vi "Alarm Playlist.vi"() -> ()   [LabVIEW 2011]
panel:
  in  "stop 3":bool
  out "Thief Alarm 2":bool
  in  "stop 2":bool
  out "Thief Alarm":bool
  in  "stop":bool
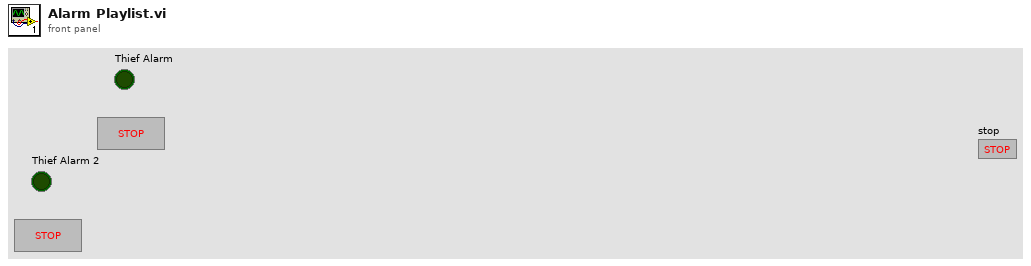
[diagram p1: front panel]
types:
  T1 = typedef "Sound Output Task ID.ctl" = u32
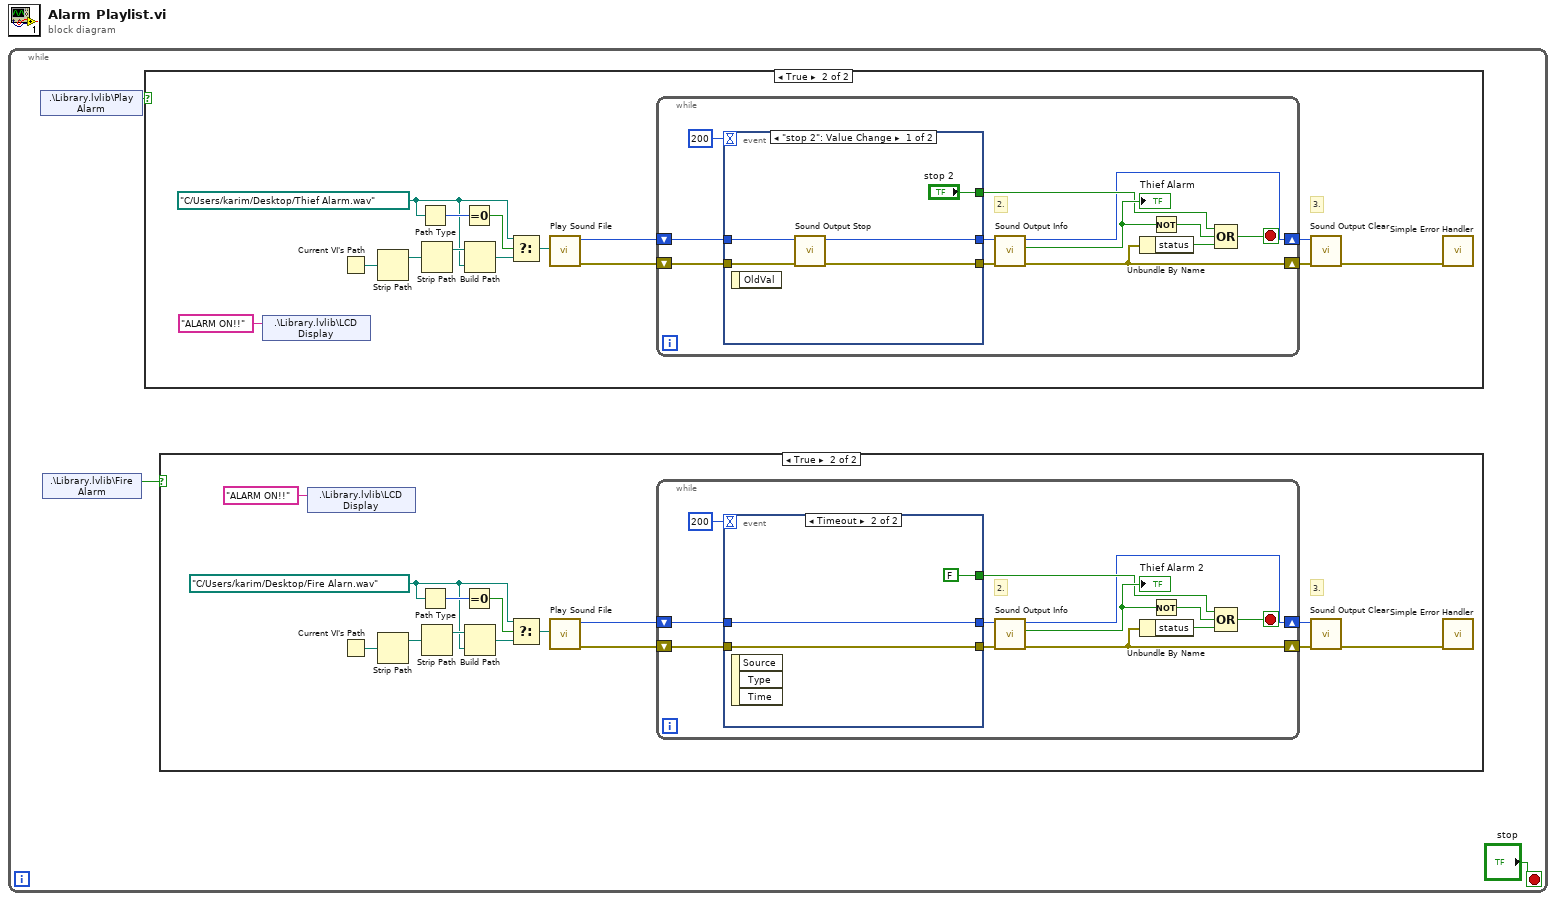
[diagram p0: block diagram]
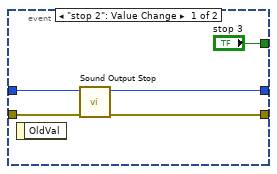
[diagram p3: hidden frame]
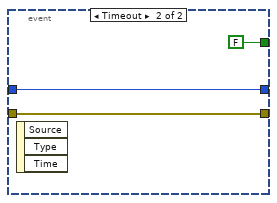
[diagram p5: hidden frame]
diagram:
  n1 = while {
    stop <- "stop" stop-if-true
    n2 = shared-variable ".\\Library.lvlib\\Play Alarm"() -> (w2:bool)  [unwired: 1 in, 1 out]
    n3 = shared-variable ".\\Library.lvlib\\Fire Alarm"() -> (w1:bool)  [unwired: 1 in, 1 out]
    n4 = case shown="True" w2 {
      frame False {
      }
      frame True {
        w39 = path "C:/Users/karim/Desktop/Thief Alarm.wav" ("Sound File Path")
        # "3."
        n5 = shared-variable ".\\Library.lvlib\\LCD Display"("ALARM ON!!" ("LCD Display")) -> ()  [unwired: 1 in, 1 out]
        n6 = Current VI's Path() -> (path=w42:path)
        n7 = Strip Path(path=w42) -> (stripped path=w41:path)  [unwired: 1 out]
        n8 = Path Type(1:w39) -> (0:w46:i16)
        n9 = Strip Path(path=w41) -> (stripped path=w40:path)  [unwired: 1 out]
        n10 = Equal To 0?(x=w46) -> (x = 0?=w45:bool)
        n11 = Build Path(base path=w40, name or relative path=w39) -> (appended path=w44:path)
        n12 = Select(t=w39, s=w45, f=w44) -> (s? t:f=w43:path)
        n13 = call <vilib>:"Play Sound File.vi"("path"=w43) -> ("error out"=w50:errorcluster, "task ID"=w51:T1)  [unwired: 9 in]
        n14 = while {
          shift-right: [w52] -> w49
          shift-left: w50 -> [w61]
          shift-right: [w54] -> w48
          shift-left: w51 -> [w62]
          stop <- w55 stop-if-true
          # "2."
          n15 = event shown="[0] \"stop 2\": Value Change" {
            selector: _ -> [_ _]
            dyn-events: _ -> [_ _]
            timeout: 200 -> [_ _]
            tunnel: w61 -> [w68 w70]
            tunnel: [w67 w70] -> w60
            tunnel: w62 -> [w66 w71]
            tunnel: [w65 w71] -> w53
            tunnel: ["stop 2" FALSE ("Stop")] -> w56
            event "stop 2": Value Change {
              n16 = event-data() -> ()  [unwired: 1 in, 1 out]
              n17 = call <vilib>:"Sound Output Stop.vi"("error in (no error)"=w68, "task ID"=w66) -> ("error out"=w67:errorcluster, "task ID out"=w65:T1)  [unwired: 8 in]
            }
            event Timeout {
              n18 = event-data() -> ()  [unwired: 1 in, 3 out]
            }
          }
          n19 = call <vilib>:"Sound Output Info.vi"("error in (no error)"=w60, "task ID"=w53) -> ("error out"=w52:errorcluster, "is playing?"=w59:bool, "task ID out"=w54:T1)  [unwired: 6 in, 1 out]
          "Thief Alarm" <- w59
          n20 = Unbundle By Name(w52) -> ("status"=w58:bool)
          n21 = Not(x=w59) -> (.not. x?=w57:bool)
          n22 = Compound Arithmetic op=OR(w56, w57, w58) -> (w55:bool)
        }
        n23 = call <vilib>:"Sound Output Clear.vi"("error in (no error)"=w49, "task ID"=w48) -> ("error out"=w47:errorcluster)  [unwired: 9 in]
        n24 = call <vilib>:"Simple Error Handler.vi"("error in (no error)"=w47) -> ()  [unwired: 4 in, 5 out]
      }
    }
    n25 = case shown="True" w1 {
      frame False {
      }
      frame True {
        w5 = path "C:/Users/karim/Desktop/Fire Alarn.wav" ("path")
        # "3."
        n26 = shared-variable ".\\Library.lvlib\\LCD Display"("ALARM ON!!" ("LCD Display")) -> ()  [unwired: 1 in, 1 out]
        n27 = Current VI's Path() -> (path=w8:path)
        n28 = Strip Path(path=w8) -> (stripped path=w7:path)  [unwired: 1 out]
        n29 = Path Type(1:w5) -> (0:w12:i16)
        n30 = Strip Path(path=w7) -> (stripped path=w6:path)  [unwired: 1 out]
        n31 = Equal To 0?(x=w12) -> (x = 0?=w11:bool)
        n32 = Build Path(base path=w6, name or relative path=w5) -> (appended path=w10:path)
        n33 = Select(t=w5, s=w11, f=w10) -> (s? t:f=w9:path)
        n34 = call <vilib>:"Play Sound File.vi"("path"=w9) -> ("error out"=w16:errorcluster, "task ID"=w17:T1)  [unwired: 9 in]
        n35 = while {
          shift-right: [w18] -> w15
          shift-left: w16 -> [w27]
          shift-right: [w20] -> w14
          shift-left: w17 -> [w28]
          stop <- w21 stop-if-true
          # "2."
          n36 = event shown="[1] Timeout" {
            selector: _ -> [_ _]
            dyn-events: _ -> [_ _]
            timeout: 200 -> [_ _]
            tunnel: w27 -> [w34 w36]
            tunnel: [w33 w36] -> w26
            tunnel: w28 -> [w32 w37]
            tunnel: [w31 w37] -> w19
            tunnel: ["stop 3" FALSE ("Stop")] -> w22
            event "stop 2": Value Change {
              n37 = event-data() -> ()  [unwired: 1 in, 1 out]
              n38 = call <vilib>:"Sound Output Stop.vi"("error in (no error)"=w34, "task ID"=w32) -> ("error out"=w33:errorcluster, "task ID out"=w31:T1)  [unwired: 8 in]
            }
            event Timeout {
              n39 = event-data() -> ()  [unwired: 1 in, 3 out]
            }
          }
          n40 = call <vilib>:"Sound Output Info.vi"("error in (no error)"=w26, "task ID"=w19) -> ("error out"=w18:errorcluster, "is playing?"=w25:bool, "task ID out"=w20:T1)  [unwired: 6 in, 1 out]
          "Thief Alarm 2" <- w25
          n41 = Unbundle By Name(w18) -> ("status"=w24:bool)
          n42 = Not(x=w25) -> (.not. x?=w23:bool)
          n43 = Compound Arithmetic op=OR(w22, w23, w24) -> (w21:bool)
        }
        n44 = call <vilib>:"Sound Output Clear.vi"("error in (no error)"=w15, "task ID"=w14) -> ("error out"=w13:errorcluster)  [unwired: 9 in]
        n45 = call <vilib>:"Simple Error Handler.vi"("error in (no error)"=w13) -> ()  [unwired: 4 in, 5 out]
      }
    }
  }
